vi "Focus Move Relative.vi"(8 "error in (no error)":errorcluster, 9 "Counts":i32, 10 "Motor (0:n-1)":i32, 11 "NewFocus in":refnum<class "NewFocus.lvclass">) -> (0 "error out":errorcluster, 2 "response":string, 3 "NewFocus out":refnum<class "NewFocus.lvclass">)   [LabVIEW 2024, in "NewFocus.lvclass"]
uses:
  NewFocus.lvclass
  NewFocus.lvclass/NewFocus.ctl
  Focus Class/Focus Class.lvclass
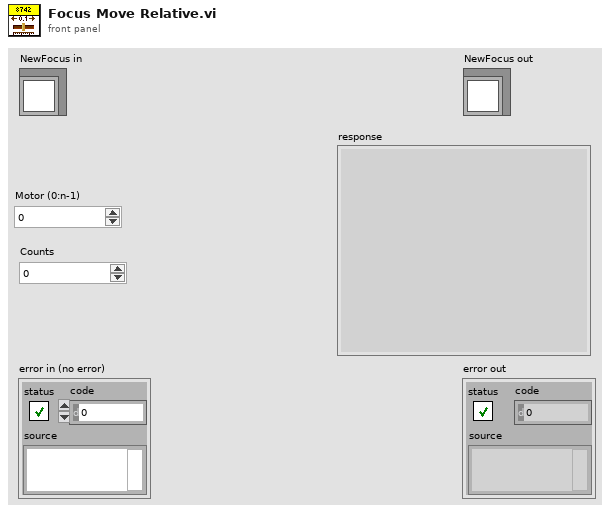
[diagram p1: front panel]
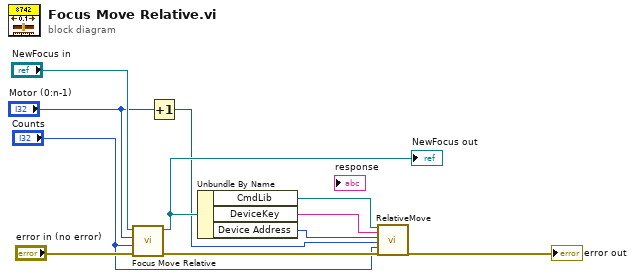
[diagram p0: block diagram]
diagram:
  n1 = call-parent "Focus Move Relative.vi"("error in (no error)"="error in (no error)", "Counts"="Counts", "Motor (0:n-1)"="Motor (0:n-1)", "Focus Class in"="NewFocus in") -> ("error out"=w9:errorcluster, "Focus Class out"=w2:refnum<class "NewFocus.lvclass">)  [unwired: 5 in, 1 out]
  "NewFocus out" <- w2
  n2 = Increment(x="Motor (0:n-1)") -> (x+1=w1:i32)
  n3 = Unbundle By Name(w2) -> ("CmdLib"=w8:refnum<k24>, "DeviceKey"=w7:string, "Device Address"=w6:i32)
  n4 = call "RelativeMove.vi"("CmdLib In"=w8, "DeviceKey In"=w7, "Device Address In"=w6, "Motor"=w1, "Relative Steps"="Counts", "error in (no error)"=w9) -> ("error out"=→"error out":errorcluster)  [unwired: 10 in, 3 out]
